vi "AcquireHardware.vi"(8 "error in (no error)":errorcluster, 11 "ThorLabsCsCamera in":refnum<class "ThorLabsCsCamera.lvclass">) -> (0 "error out":errorcluster, 2 "Image Out":T1(plugin-control), 3 "ThorLabsCsCamera out":refnum<class "ThorLabsCsCamera.lvclass">)   [LabVIEW 2020, in "ThorLabsCsCamera.lvclass"]
uses:
  ThorLabsCsCamera.lvclass
  C:/GEECS/Developers Version/source/Device Drivers/Point Grey Camera/Point Grey Camera.lvclass
  ThorLabsCsCamera.lvclass/ThorLabsCsCamera.ctl
  Point Grey Camera/Point Grey Camera.lvclass/Point Grey Camera.ctl
  C:/GEECS/Developers Version/source/Device Drivers/Point Grey Camera/Library_X86/Thorlabs.TSI.TLCameraInterfaces.dll
  Point Grey Camera/Library_X86/Thorlabs.TSI.TLCameraInterfaces.dll
  C:/GEECS/Developers Version/source/Device Drivers/Point Grey Camera/Library_X86/Thorlabs.TSI.ImageDataInterfaces.dll
  Point Grey Camera/Library_X86/Thorlabs.TSI.ImageDataInterfaces.dll
  Point Grey Camera/Read Image ref.vi
  Point Grey Camera/Read Settings 2.vi
panel:
  out "acq time (ms)":u32
  out "Intensity Graph Mono":u16[][](graph)
  out "FrameNumber":u32
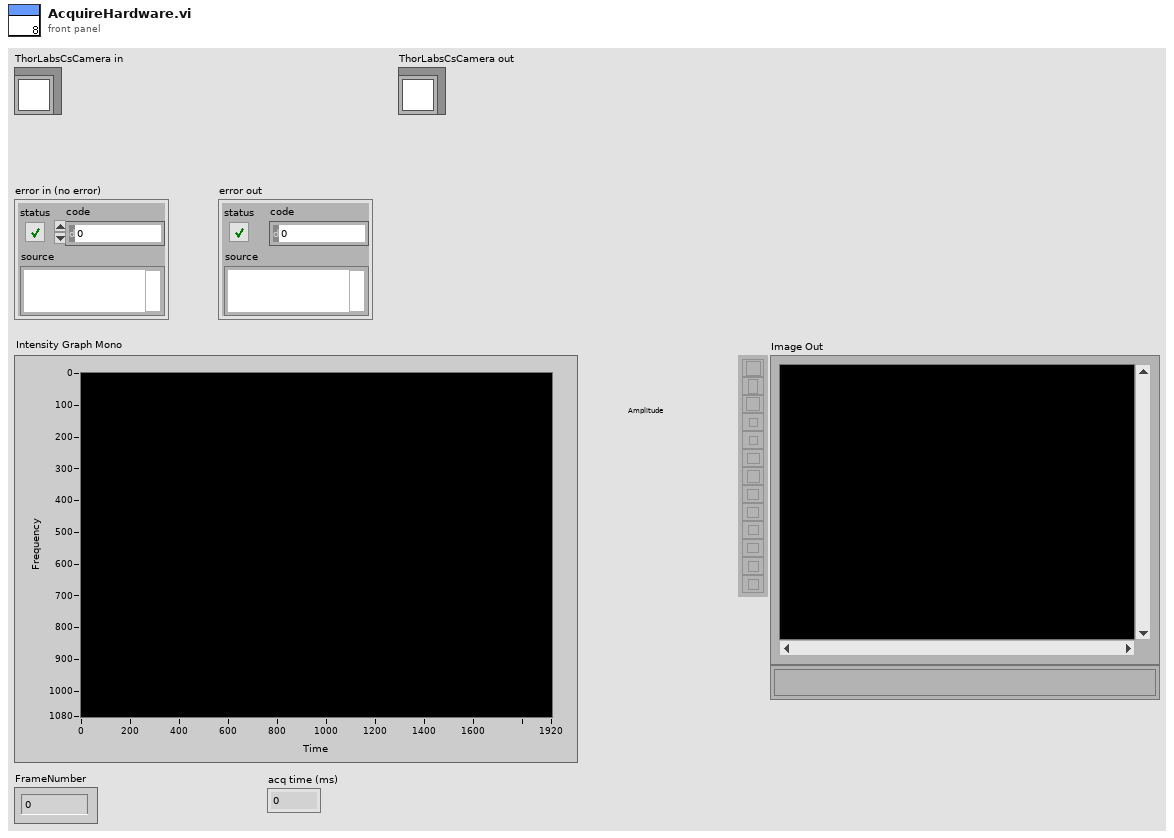
[diagram p1: front panel]
types:
  T1 = typedef "IMAQ Image.ctl" = refnum<image>
  T2 = typedef "Point Grey Camera.lvclass/SettingsTypdef.ctl" = cluster{"Trigger":T3, "Gain":cluster{"Value":dbl, "Min":dbl, "Max":dbl, "StepSize":dbl, "Tolerance":dbl, "valueactual":dbl}, "Exposure":cluster{"Value":dbl, "Min":dbl, "Max":dbl, "StepSize":dbl, "Tolerance":dbl, "valueactual":dbl}, "Timeout":cluster{"Value":dbl, "Min":dbl, "Max":dbl, "StepSize":dbl, "Tolerance":dbl, "valueactual":dbl}, "LocalSavingPath":path, "Save":T3, "TriggerDelay":cluster{"Value":dbl, "Min":dbl, "Max":dbl, "StepSize":dbl, "Tolerance":dbl, "valueactual":dbl}, "CamSession":string, "ROI":T4, "MaxGUIPixel":cluster{"Value":dbl, "Min":dbl, "Max":dbl, "StepSize":dbl, "Tolerance":dbl, "valueactual":dbl}, "Target":cluster{"X":cluster{"Value":dbl, "Min":dbl, "Max":dbl, "StepSize":dbl, "Tolerance":dbl, "valueactual":dbl}, "Y":cluster{"Value":dbl, "Min":dbl, "Max":dbl, "StepSize":dbl, "Tolerance":dbl, "valueactual":dbl}}, "Analysis":T3, "maxshot#":dbl, "SpatialCalibration":cluster{"Value":dbl, "Min":dbl, "Max":dbl, "StepSize":dbl, "Tolerance":dbl, "valueactual":dbl}, "roistatus":T3, "Lineout":T3, "AnalysisThreshold":cluster{"Value":dbl, "Min":dbl, "Max":dbl, "StepSize":dbl, "Tolerance":dbl, "valueactual":dbl}, "TargetSize":cluster{"X":cluster{"Value":dbl, "Min":dbl, "Max":dbl, "StepSize":dbl, "Tolerance":dbl, "valueactual":dbl}, "Y":cluster{"Value":dbl, "Min":dbl, "Max":dbl, "StepSize":dbl, "Tolerance":dbl, "valueactual":dbl}}, "Simulation":T3, "SpatialCalibrationY":cluster{"Value":dbl, "Min":dbl, "Max":dbl, "StepSize":dbl, "Tolerance":dbl, "valueactual":dbl}, "Target2":cluster{"X":cluster{"Value":dbl, "Min":dbl, "Max":dbl, "StepSize":dbl, "Tolerance":dbl, "valueactual":dbl}, "Y":cluster{"Value":dbl, "Min":dbl, "Max":dbl, "StepSize":dbl, "Tolerance":dbl, "valueactual":dbl}}, "Target2Size":cluster{"X":cluster{"Value":dbl, "Min":dbl, "Max":dbl, "StepSize":dbl, "Tolerance":dbl, "valueactual":dbl}, "Y":cluster{"Value":dbl, "Min":dbl, "Max":dbl, "StepSize":dbl, "Tolerance":dbl, "valueactual":dbl}}, "Crosshair":cluster{"Label1":string, "Label2":string}, "Max2ndMomRadius":cluster{"Value":dbl, "Min":dbl, "Max":dbl, "StepSize":dbl, "Tolerance":dbl, "valueactual":dbl}, "SaveType":T5, "BackgroundPath":path, "GUI8bit":T3, "GUICompression":T3, "CompressionQuality":cluster{"Value":dbl, "Min":dbl, "Max":dbl, "StepSize":dbl, "Tolerance":dbl, "valueactual":dbl}, "SaveAsync":T3, "PerspectivePath":path, "PerspectiveCorrectGUI":T3, "BlackLevel":cluster{"Value":dbl, "Min":dbl, "Max":dbl, "StepSize":dbl, "Tolerance":dbl, "valueactual":dbl}, "TargetBP":cluster{"X":cluster{"Value":dbl, "Min":dbl, "Max":dbl, "StepSize":dbl, "Tolerance":dbl, "valueactual":dbl}, "Y":cluster{"Value":dbl, "Min":dbl, "Max":dbl, "StepSize":dbl, "Tolerance":dbl, "valueactual":dbl}}, "PythonAnalysis":T3, "PythonFunctionName":string, "PythonLineout":T3, "PythonVersion":string, "GEECSBuildsPath":path, "DisplayPythonProcessedImage":T3, "PythonModuleName":string, "AnalysisThresholdHigh":cluster{"Value":dbl, "Min":dbl, "Max":dbl, "StepSize":dbl, "Tolerance":dbl, "valueactual":dbl}, "AnalysisMedianRank":cluster{"Value":dbl, "Min":dbl, "Max":dbl, "StepSize":dbl, "Tolerance":dbl, "valueactual":dbl}, "ClockSpeed":cluster{"Value":dbl, "Min":dbl, "Max":dbl, "StepSize":dbl, "Tolerance":dbl, "valueactual":dbl}, "AutoTrigger":T3, "AutoTriggerLevelMeanCounts":cluster{"Value":dbl, "Min":dbl, "Max":dbl, "StepSize":dbl, "Tolerance":dbl, "valueactual":dbl}, "AnalysisROILeft":cluster{"Value":dbl, "Min":dbl, "Max":dbl, "StepSize":dbl, "Tolerance":dbl, "valueactual":dbl}, "AnalysisROIRight":cluster{"Value":dbl, "Min":dbl, "Max":dbl, "StepSize":dbl, "Tolerance":dbl, "valueactual":dbl}, "AnalysisROITop":cluster{"Value":dbl, "Min":dbl, "Max":dbl, "StepSize":dbl, "Tolerance":dbl, "valueactual":dbl}, "AnalysisROIBottom":cluster{"Value":dbl, "Min":dbl, "Max":dbl, "StepSize":dbl, "Tolerance":dbl, "valueactual":dbl}, "AnalysisROI":T3, "UseSoftwareTrigger":T3, "UDPtrigger":T3, "AutoTriggerLevelMaxCounts":cluster{"Value":dbl, "Min":dbl, "Max":dbl, "StepSize":dbl, "Tolerance":dbl, "valueactual":dbl}}
  T3 = typedef "OnOffTypeDef.ctl" = enum16{"off", "on"}
  T4 = typedef "ROI_TypDef.ctl" = cluster{"Width":cluster{"Value":dbl, "Min":dbl, "Max":dbl, "StepSize":dbl, "Tolerance":dbl, "valueactual":dbl}, "Height":cluster{"Value":dbl, "Min":dbl, "Max":dbl, "StepSize":dbl, "Tolerance":dbl, "valueactual":dbl}, "OffsetX":cluster{"Value":dbl, "Min":dbl, "Max":dbl, "StepSize":dbl, "Tolerance":dbl, "valueactual":dbl}, "OffsetY":cluster{"Value":dbl, "Min":dbl, "Max":dbl, "StepSize":dbl, "Tolerance":dbl, "valueactual":dbl}}
  T5 = typedef "Image save type.ctl" = enum16{"PNG", "BMP", "JPEG", "TDMS", "hdf5"}
  T6 = enum32{"Invalid", "Standard", "Closed", "Hidden", "Minimized", "Maximized"}
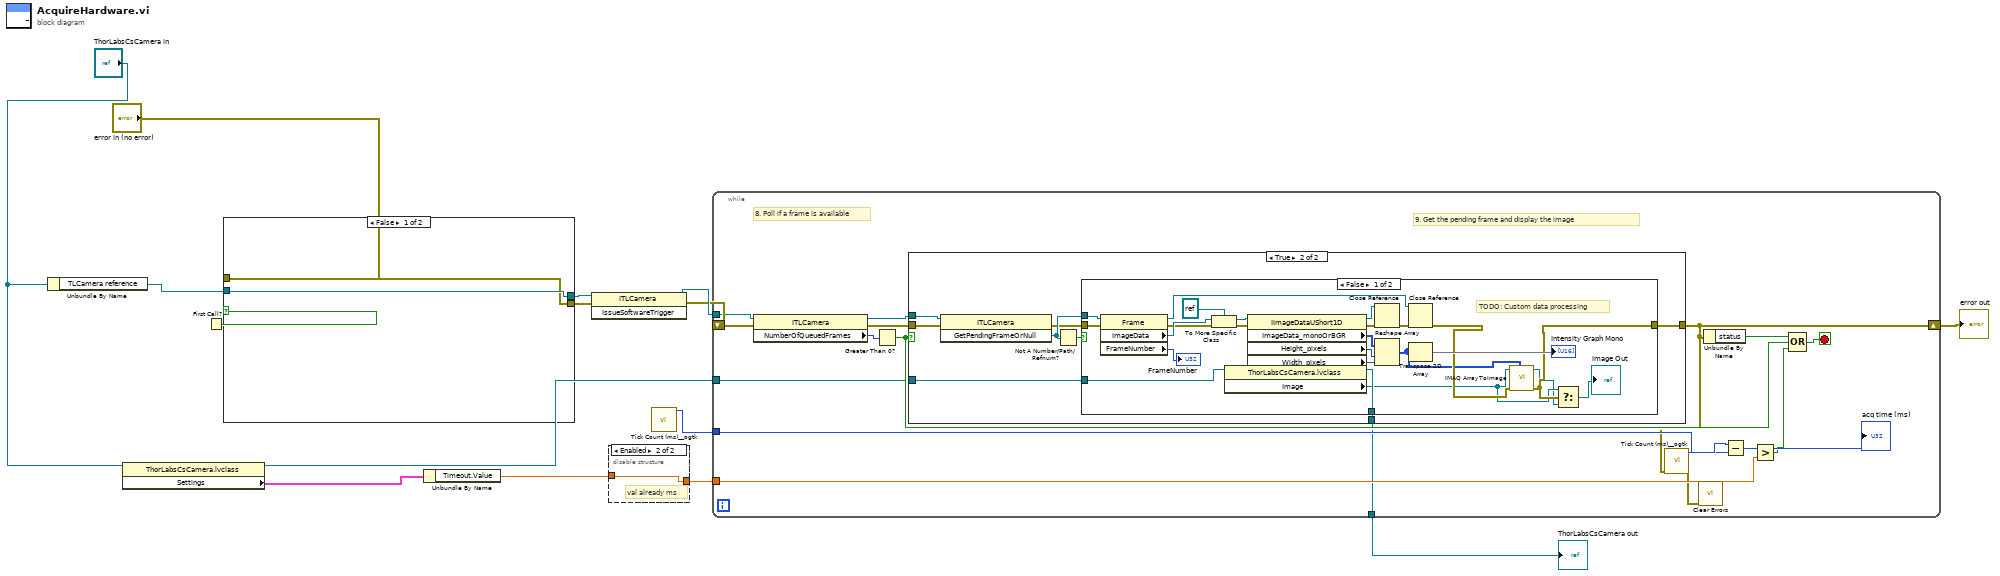
[diagram p0: block diagram]
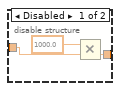
[diagram p2: hidden frame]
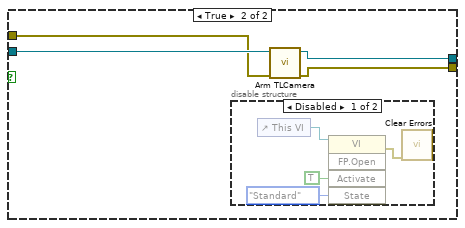
[diagram p5: hidden frame]
diagram:
  n1 = Unbundle By Name("ThorLabsCsCamera in") -> ("TLCamera reference"=w14:refnum<k24>)
  n2 = property class="ThorLabsCsCamera.lvclass"(reference="ThorLabsCsCamera in") -> (reference out=w7:refnum<class "ThorLabsCsCamera.lvclass">, "Settings"=w10:T2)  [unwired: 1 in, 1 out]
  n3 = First Call?() -> (First Call?: T/F=w15:bool)
  n4 = case shown="False" w15 {
    tunnel: w14 -> [w17 w21]
    tunnel: "error in (no error)" -> [w16 w20]
    tunnel: [w17 w19] -> w4
    tunnel: [w16 w18] -> w3
    frame False {
    }
    frame True {
      n5 = disable-structure shown="Disabled" {
        frame Disabled {
          n6 = control-ref of="This VI"() -> (w25:refnum<vi>)
          n7 = invoke class="VI" method="FP.Open"(reference=w25, "Activate"=TRUE ("Activate?"), "State"=T6."Standard") -> (error out=w22:errorcluster)  [unwired: 2 in, 4 out]
          n8 = call <vilib>:"Clear Errors.vi"("error in (no error)"=w22) -> ()  [unwired: 5 in, 2 out]
        }
        frame Enabled {
        }
      }
      n9 = call "Arm TLCamera.vi"("error in (no error)"=w20, "TLCamera reference"=w21) -> ("error out"=w18:errorcluster, "TLCamera reference out"=w19:refnum<k24>)  [unwired: 8 in]
    }
  }
  n10 = Unbundle By Name(w10) -> ("Timeout.Value"=w9:dbl)
  n11 = invoke class="ITLCamera" method="IssueSoftwareTrigger"(reference=w4, error in=w3) -> (reference out=w2:refnum<k24>, error out=w1:errorcluster)  [unwired: 1 in, 1 out]
  n12 = disable-structure shown="Enabled" {
    disable-tunnel: w9 -> [w28 w29]
    disable-tunnel: [w27 w29] -> w8
    frame Disabled {
      n13 = Multiply(x=1000.0, y=w28) -> (x*y=w27:dbl)
    }
    frame Enabled {
      # "val already ms"
    }
  }
  n14 = call <userlib>:"Tick Count (ms)__ogtk.vi"() -> ("millisecond timer value"=w12:u32)  [unwired: 10 in, 1 out]
  n15 = while {
    tunnel: w2 -> [w46]
    shift-right: [w31] -> w5
    shift-left: w1 -> [w45]
    tunnel: w12 -> [w37]
    tunnel: w8 -> [w35]
    tunnel: w7 -> [w33]
    tunnel: [w32] -> w6
    stop <- w40 stop-if-true
    # "9. Get the pending frame and display the image"
    # "8. Poll if a frame is available"
    n16 = property class="ITLCamera"(reference=w46, error in=w45) -> (reference out=w42:refnum<k24>, error out=w43:errorcluster, "NumberOfQueuedFrames"=w44:i32)
    n17 = Greater Than 0?(x=w44) -> (x > 0?=w39:bool)
    n18 = case shown="True" w39 {
      tunnel: w43 -> [w48 w55]
      tunnel: w42 -> [_ w56]
      tunnel: [w48 w51] -> w31
      tunnel: w33 -> [w47 w50]
      tunnel: [w47 w49] -> w32
      frame False {
      }
      frame True {
        n19 = invoke class="ITLCamera" method="GetPendingFrameOrNull"(reference=w56, error in=w55) -> (error out=w52:errorcluster, "GetPendingFrameOrNull"=w53:refnum<k24>)  [unwired: 1 in, 1 out]
        n20 = Not A Number/Path/Refnum?(number/path/refnum=w53) -> (NaN/Path/Refnum?=w54:bool)
        n21 = case shown="False" w54 {
          tunnel: w53 -> [w71 _]
          tunnel: w52 -> [w79 w82]
          tunnel: [w60 w82] -> w51
          tunnel: w50 -> [w61 w81]
          tunnel: [w65 w81] -> w49
          frame False {
            # "TODO: Custom data processing"
            n22 = property class="Frame"(reference=w71, error in=w79) -> (reference out=w76:refnum<k24>, error out=w69:errorcluster, "ImageData"=w70:refnum<k24>, "FrameNumber"=→"FrameNumber":u32)
            n23 = To More Specific Class(target class=refnum<k24> refnum, reference=w70, error in=w69) -> (specific class reference=w67:refnum<k24>, error out=w68:errorcluster)
            n24 = property class="ThorLabsCsCamera.lvclass"(reference=w61) -> (reference out=w65:refnum<class "ThorLabsCsCamera.lvclass">, "Image"=w59:T1)  [unwired: 1 in, 1 out]
            n25 = property class="IImageDataUShort1D"(reference=w67, error in=w68) -> (reference out=w77:refnum<k24>, error out=w78:errorcluster, "ImageData_monoOrBGR"=w80:u16[], "Height_pixels"=w72:i32, "Width_pixels"=w73:i32)
            n26 = Close Reference(reference=w77, error in (no error)=w78) -> (error out=w75:errorcluster)
            n27 = Reshape Array(w80, w72, w73) -> (w62:u16[][])
            n28 = Close Reference(reference=w76, error in (no error)=w75) -> (error out=w63:errorcluster)
            n29 = Transpose 2D Array(2D array=w62) -> (transposed array=→"Intensity Graph Mono":u16[][])
            n30 = call "IMAQ ArrayToImage"("Image Pixels (U16)"=w62, "error in (no error)"=w63, "Image"=w59) -> ("error out"=w60:errorcluster, "Image Out"=w58:T1)  [unwired: 7 in]
            n31 = Select(t=w59, s=w60, f=w58) -> (s? t:f=→"Image Out":T1)
          }
          frame True {
          }
        }
      }
    }
    n32 = call <userlib>:"Tick Count (ms)__ogtk.vi"("error in (no error)"=w31) -> ("error out"=w30:errorcluster, "millisecond timer value"=w38:u32)  [unwired: 9 in]
    n33 = call <vilib>:"Clear Errors.vi"("error in (no error)"=w30) -> ()  [unwired: 5 in, 2 out]
    n34 = Unbundle By Name(w31) -> ("status"=w41:bool)
    n35 = Subtract(x=w38, y=w37) -> (x-y=w36:u32)
    "acq time (ms)" <- w36
    n36 = Greater?(x=w36, y=w35) -> (0:w34:bool)
    n37 = Compound Arithmetic op=OR(w41, w39, w34) -> (w40:bool)
  }
  "error out" <- w5
  "ThorLabsCsCamera out" <- w6
